vi "Process All FTC Functions.vi"(11 "NXT":T1={"Hardware"="NXT", "Flattened String"=""}) -> (3 "NXT":T1={"Hardware"="NXT", "Flattened String"=""})   [LabVIEW 2010, in "FTC.lvlib"]
uses:
  FTC.lvlib
  <vilib>/NXT/Subs/LVHSConnector.ctl
  Remote Interface/Remote Interface.lvlib
  CLIB/CRef/CRef.lvlib
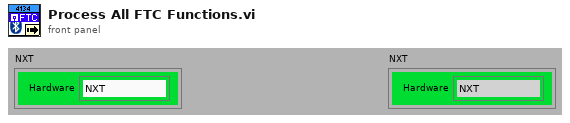
[diagram p1: front panel]
types:
  T1 = typedef "LVHSConnector.ctl" = cluster{"Hardware":string, "Flattened String":string}
  T2 = cluster{"Controller 1":string, "Controller 2":string, "Stopped?":bool, "Online?":bool, "Packet Received?":bool, "Teleop?":bool, "Enabled?":enum16{"Disabled", "Enabled"}}
  T3 = typedef "CRef.lvlib/Boolean CReference.ctl" = cluster{"Boolean CRef Address":u16, "Type":enum8{"Null", "Boolean", "U8", "I8", "U16", "I16", "U32", "I32", "U64", "I64", "Single", "Double", "Extended", "CSG", "CDB", "CXT", "Boolean(Def)"}}
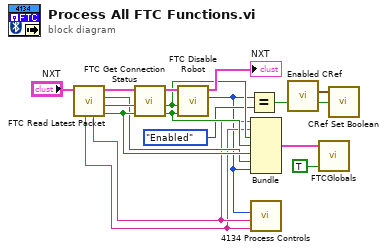
[diagram p0: block diagram]
diagram:
  n1 = call <vilib>:"FTC Read Latest Packet.vi"("NXT"="NXT") -> ("Packet Received?"=w9:bool, "Stopped?"=w17:bool, "Teleop?"=w8:bool, "NXT"=w14:T1, "Controller 1"=w6:string, "Controller 2"=w5:string)  [unwired: 5 in]
  n2 = call <vilib>:"FTC Get Connection Status.vi"("Packet Received?"=w9, "Stopped?"=w17, "NXT"=w14) -> ("Online?"=w10:bool, "Stopped?"=w11:bool, "NXT"=w13:T1)  [unwired: 5 in]
  n3 = call <vilib>:"FTC Disable Robot.vi"("Online?"=w10, "Stopped?"=w11, "NXT"=w13) -> ("Enabled?"=w1:enum16{"Disabled", "Enabled"}, "NXT"=→"NXT":T1)  [unwired: 3 in]
  n4 = Equal?(x=w1, y=enum16{"Disabled", "Enabled"}."Enabled") -> (x = y?=w2:bool)
  n5 = Bundle("Controller 1"=w6, "Controller 2"=w5, "Stopped?"=w11, "Online?"=w10, "Packet Received?"=w9, "Teleop?"=w8, "Enabled?"=w1) -> (w7:T2)  [unwired: 1 in]
  n6 = call "4134 Process Controls.vi"("Remote 2 Packet"=w5, "Remote 1 Packet"=w6, "Enabled? (Default)"=w1) -> ()  [unwired: 6 in, 3 out]
  n7 = call "Enabled CRef.vi"() -> ("Enabled: CRef"=w3:T3)  [unwired: 10 in]
  n8 = call "FTCGlobals.vi"("Write?"=TRUE, "Write Globals"=w7) -> ()  [unwired: 2 in, 1 out]
  n9 = call "CRef Set Boolean.vi"("Value"=w2, "Boolean CReference"=w3) -> ()  [unwired: 3 in, 1 out]
